vi "AlliGator Source Image ROI Manager.vi"() -> ()   [LabVIEW 2021, in "AlliGator ROIs.lvlib"]
doc: "Source Image ROI list display UI."
uses:
  AlliGator ROIs.lvlib
  AlliGator ROI Manager Actions.ctl
  AlliGator Refnums List.ctl
  Image/Image Control Refnum.ctl
  Image/Image Display Event.ctl
  <vilib>/Utility/miscctls.llb/LVPoint32TypeDef.ctl
  AlliGator Q Element.ctl
  AlliGator Q Event.ctl
  Variant/Variant to Data/Variant to String.vi
  AlliGator Source Image ROI Storage [SGL] v3.vi
  Image/Image.lvlib
  AlliGator Action Engine.lvlib
  Notebook/Notebook.lvlib
  AlliGator Notebook.lvlib
  Variant/Variant to Data/Variant to Data.lvlib
  AlliGator Source Image.lvlib
  AlliGator Globals, Variables & Constants.lvlib
  Rich Text Box/Rich Text Box.lvlib
panel:
  in  "ROI":i32
  out "# ROIs":i32
  in  "ROI List":i32(listbox)
  # "of"
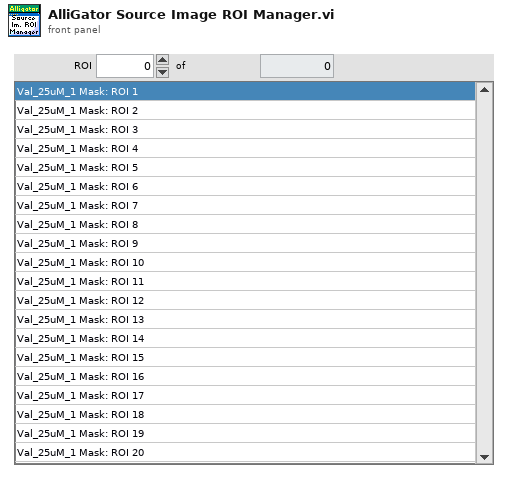
[diagram p1: front panel]
types:
  T1 = typedef "Image.lvlib/Image Control Refnum.ctl" = refnum<vi>
  T2 = typedef "AlliGator Globals, Variables & Constants.lvlib/AlliGator Refnums List.ctl" = enum16{"---------- AlliGator Controls ----------", "AlliGator Tab Control Refnum", "---------- AlliGator Indicators ----------", "Source Image Display Refnum", "Phasor Plot Display Refnum", "Decay Fit Parameter Map Refnum", "---------- AlliGator VIs ----------", "AlliGator Settings Refnum", "AlliGator Launcher Refnum"}
  T3 = typedef "AlliGator ROIs.lvlib/AlliGator ROI Manager Actions.ctl" = enum16{"Undefined", "Delete Current ROI", "Delete All Unselected ROIs", "Delete Multiple ROIs", "Delete All ROIs", "Swap ROIs", "Insert ROI", "Update Current ROI Descriptor", "Rename Current ROI", "Store New ROI", "Store Multiple ROIs", "Select Next ROI", "Select Previous ROI", "Find Selected ROI", "Show All ROIs", "Update ROI Manager Window", "Merge All ROIs", "Unmerge ROI", "Set Selected ROI by ID"}
  T4 = typedef "AlliGator ROIs.lvlib/AlliGator Image ROI Event refnum.ctl" = refnum<user-event>
  T5 = typedef "ROI Descriptor" = cluster{"Global Rectangle":i32[], "Contours":cluster{"ID":enum32{"External", "Internal"}, "Type":u32, "Coordinates":i32[]}[]}
  T6 = typedef "Image.lvlib/Image Display Event.ctl" = cluster{"Item Tag":string, "Image Control Refnum":T1, "Coords":T7, "Item Path":string}
  T7 = typedef "LVPoint32TypeDef.ctl" = cluster{"Horizontal":i32, "Vertical":i32}
  T8 = typedef "AlliGator Action Engine.lvlib/AlliGator Q Element.ctl" = cluster{"AlliGator Q Event":T9, "Data":variant}
  T9 = typedef "AlliGator Action Engine.lvlib/AlliGator Q Event.ctl" = enum16{"---- Files ----", "Files:Set Batch Export Files To Save", "Files:Set Dataset Loading & Pre-processing Options", "Files:Check #Frames in Dataset", "Files:Increment Frame Index", "Files:Open Mask Image", "Files:Open White Light Image", "Files:Open Single Dataset", "Files:New Folder of Folders Selected", "Files:Load File (all Types)_Scriptable", "Files:Move Flattened Series to Folders Series", "Files:Select Folder", "Files:Load FLI Dataset", "Files:Load Swiss SPAD 1 Dataset", "Files:Load Swiss SPAD 2 Dataset", "Files:Load .sdt FLI Dataset", "Files:Load .ptu FLI Dataset", "Files:Load .bin FLI Dataset", "Files:Load Single Gate Image Folder", "Files:Load I/m/phi Dataset (deprecated)", "Files:Load Single Image", "Files:Subtract Background File", "Files:Export FLI Dataset", "Files:Load HDF5 FLI Dataset", "Files:Set Destination File Path", "Files:Save Mask Image", "Files:Batch Conversion", "Files:New Folder Selected", "Files:Close FLI Dataset", "Files:Close FLI Dataset Series", "Files:Close White Light Image", "Files:Close Mask Image", "---- FLI Dataset ----", "FLI Dataset:Channel Arithmetic", "FLI Dataset:Export Average Lifetime Map as ASCII", "FLI Dataset:Export User-Defined Quantity Map as ASCII", "FLI Dataset:Python Function FLI Dataset Event", "FLI Dataset:ROI Analysis", "FLI Dataset:Tilted Logistic Square Gated IRF Characteristics Map", "FLI Dataset:Logistic Square Gated IRF Characteristics Map", "FLI Dataset:Square Gated IRF Characteristics Map", "FLI Dataset:Multi-ROI Single-Pixel Phasor Analysis", "FLI Dataset:Multi-ROI Single-Pixel NLSF Analysis", "FLI Dataset:All ROIs IRF Extraction", "FLI Dataset:All ROIs Decay Fit Non-Interactive (Fast + Individual IRF)", "FLI Dataset:All ROIs Phasor Analysis", "FLI Dataset:All ROIs Decay Fit", "FLI Dataset:Fluorescence Decay Statistics", "FLI Dataset:Update Decay Statistics Graph", "FLI Dataset:Get Decay from ROI", "FLI Dataset:All ROIs Average Lifetimes", "---- FLI Dataset Series ----", "FLI Dataset Series:Sum All Datasets in Series", "FLI Dataset Series:Add Dataset to Accumulated Dataset", "FLI Dataset Series:Display Accumulated Dataset", "FLI Dataset Series:Clear Dataset Series Sum", "FLI Dataset Series:Time-Series Analysis (NLSF)", "FLI Dataset Series:Time-Series Analysis (Phasor)", "---- Image ----", "Image:Update Image Profile Plots", "Image:Image Histogram Cursor Move", "Image:Image Histogram", "Image:Image Contrast", "Image:Set Image Histogram Cursor Move Flag", "Image:Clear Image Overlay", "Image:Use ROI as Search Area", "Image:Set ROI Diameter", "Image:Save Image Data as TIFF", "Image:Save Displayed Image with Overlay", "Image:Save Image Overlay Only", "Image:Save Image as Hot Pixel Mask", "Image:Change Source Image Color Palette", "Image:Copy Image to Clipboard", "Image:Source Image ROI Selection", "Image:Delete All ROIs", "Image:Delete All Unselected ROIs", "Image:Delete ROI", "Image:Merge All ROIs", "Image:Store ROI", "Image:Source Image ROI Storage", "Image:Export ROI Description to Notebook", "Image:Save ROI", "Image:Load ROI", "Image:Paste ROI Definition", "Image:Clear ROI", "Image:Identify ROIs in Mask Image", "Image:Create Complementary ROI", "Image:Create Contour ROI", "Image:Create ROI(s) from Pixels with Peak above Min_Scriptable", "Image:Create ROI(s) from Pixels with Intensity above Min_Scriptable", "Image:Compute ROI Statistics", "Image:Delete ROI(s) based on ROI Characteristics", "Image:Create ROI Grid", "Image:ROI to Individual Pixel ROIs", "Image:Python Function Source Image Event", "Image:Show Phasor Calibration Map ROI Centers", "Image:Convert ROI to Mask Image", "Image:Mouse Move", "Image:Mouse Up", "Image:Set Source Image Mouse Move Flag", "Image:Add Scale Bar Overlay", "Image:Delete Existing ROIs Option", "---- Decay ----", "Decay:Clear IRF/Reference Plot", "Decay:Clear Local IRFs", "Decay:Add Decay to Graph", "Decay:Smoothen Plot", "Decay:Smoothen Plot Tail", "Decay:Average Selected Plots", "Decay:Extract IRF", "Decay:Optimal IRF Extraction", "Decay:Threshold IRF", "Decay:Fit to Model IRF", "Decay:Fit IRF to Square Gate", "Decay:Fit IRF to Logistic Square Gate", "Decay:Fit IRF to Tilted Logistic Square Gate", "Decay:Create Bounding Cursors Set", "Decay:Export Bounding Cursors Definition to Notebook", "Decay:Denoise Plot", "Decay:Compute Cumulative Function", "Decay:Use as Reference Decay", "Decay:Show Reference Decay/IRF", "Decay:Extrapolate Decay", "Decay:Create Head & Tail Bounding Cursors", "Decay:Store Cursor-defined Head & Tail Fractions", "Decay:Rebin Plot", "Decay:1-Normalize Decay", "Decay:[0-1]-Normalize Plot", "Decay:Straighten Decay", "Decay:Shift Decay", "Decay:Fold Decay", "Decay:Fit Decay", "Decay:Global Fit of Selected Decays", "Decay:Post Global Fit Script", "Decay:Add Global Fit Parameters to Graph", "Decay:Add Decay Parameter(s) to Plot (Graph)", "Decay:Export Decay to Phasor Graph", "Decay:Plot Decay Shifts", "Decay:Compute Average Lifetime", "Decay:Plot Convolution", "Decay:Graph Tip Strip Update", "---- Decay Statistics ----", "Decay Statistics:Tip Strip Update", "---- Intensity Time Trace ----", "Intensity Time Trace:Use File Timestamp", "Intensity Time Trace:Load Intensity Corrections File", "Intensity Time Trace:Clear Intensity Corrections File", "Intensity Time Trace:Tip Strip Update", "---- Phasor Plot ----", "Phasor Plot:Build Phasor Plot", "Phasor Plot:Change Phasor Plot Color Palette", "Phasor Plot:Adjust Phasor Plot Display Range", "Phasor Plot:Highlight Image ROI in Phasor Plot", "Phasor Plot:Save Phasor Plot Image with Overlay", "Phasor Plot:Export Complex Phasor Map", "Phasor Plot:Export Phasor Ratio Map", "Phasor Plot:Export Average Lifetime Map", "Phasor Plot:Compute Phase Lifetime Histogram", "Phasor Plot:Compute Phasor Ratio Histogram", "Phasor Plot:Compute Phase Lifetime vs Intensity Scatter Plot", "Phasor Plot:Weber 2-Component Decomposition", "Phasor Plot:Update Phasor Color Map Vertices", "Phasor Plot:Clear Phasor Overlay", "Phasor Plot:Use Segment Extremities as References", "Phasor Plot:Use UC/Segment Intersections as References", "Phasor Plot:Use UC/Principal Axis Intersections as References", "Phasor Plot:Use UC/Linear Fit Intersections as References", "Phasor Plot:Update Phasor Plot Reference", "Phasor Plot:Show Local Phasor Info in Phasor Plot", "Phasor Plot:Update Phasor Plot State", "Phasor Plot:Phasor Plot ROI Storage", "Phasor Plot:Phasor Plot ROI Selection", "Phasor Plot:Python Function Phasor Plot Event", "Phasor Plot:Overlay Phasor ROI, Ratio or Map in Source Image", "Phasor Plot:Compute Decay of Selected Phasors", "Phasor Plot:Phasor at Image Pixel", "Phasor Plot:Mouse Move", "Phasor Plot:Mouse Up", "Phasor Plot:Display Range Mouse Move", "Phasor Plot:Set Mouse Move Flag", "---- Phasor Graph ----", "Phasor Graph:Calibrated Phasor Map Series", "Phasor Graph:Whole Image Phasor Scatter Plot (Todo)", "Phasor Graph:Get Phasor Value", "Phasor Graph:Create New Phasor Plot Dialog", "Phasor Graph:Update Last Phasor Value", "Phasor Graph:Update Phasor (m, phi)", "Phasor Graph:Remove Single Phasor from Plot", "Phasor Graph:Add Single Phasor to Plot", "Phasor Graph:Remove Phasor Plot", "Phasor Graph:Remove Selected Phasor Plots", "Phasor Graph:Clear Phasor Data", "Phasor Graph:Clear Phasor Graph", "Phasor Graph:Cursor Move", "Phasor Graph:Draw Cursor Connecting Line", "Phasor Graph:Clear Cursor Connecting Line", "Phasor Graph:Find UC Intersection", "Phasor Graph:Use UC/Cursor-Defined Line Intersections", "Phasor Graph:Use Selected Plots Fitted Line/UC Intersections", "Phasor Graph:Use Selected Plots Principal Axis/UC Intersections", "Phasor Graph:Show Single Phasor", "Phasor Graph:Save Single Phasor Plot", "Phasor Graph:Save All Phasor Plots", "Phasor Graph:Load Phasor Plot(s)", "Phasor Graph:Phasor Multiplication", "Phasor Graph:Compute Average Phasor", "Phasor Graph:Compute Multiple Average Phasors (Selected Plots)", "Phasor Graph:Export Single Phasor Plot Phase Lifetimes", "Phasor Graph:Phase Lifetime Trajectory", "Phasor Graph:Phase Lifetime vs Intensity Scatter Plot (deprecated)", "Phasor Graph:Parameter 2 vs Parameter 1 Scatter Plot", "Phasor Graph:Use Cursor n Location", "Phasor Graph:Set Reference n to Current Phase Lifetime Value", "Phasor Graph:Set Reference n to Lifetime Value", "Phasor Graph:Set Cursor n Location", "Phasor Graph:Save Phasor Graph Image", "Phasor Graph:Update SEPL Plot", "Phasor Graph:Export Single Phasor Plot Data", "Phasor Graph:Export Selected Phasor Plots Data", "Phasor Graph:Python Function Phasor Graph Event", "Phasor Graph:Tip Strip Update", "---- Calibration ----", "Calibration:Set Calibration Type", "Calibration:Load/Save Phasor Calibration", "Calibration:Load/Save Phasor Calibration Series", "Calibration:Load/Save Phasor Calibration Map", "Calibration:Use as Calibration", "Calibration:Compute Optimal Calibration from Phasor References", "Calibration:Clear Phasor Calibration", "Calibration:Single Phasor Calibration Information", "Calibration:Use as Calibration Series", "Calibration:Use as Calibration Map", "Calibration:Clear Calibration Series", "Calibration:Phasor Calibration Series Information", "Calibration:Clear Calibration Map", "Calibration:Phasor Calibration Map Information", "Calibration:Apply Phasor Calibration", "Calibration:Update Single Plot Calibration", "Calibration:Update Multiple Plots Calibration", "Calibration:Clear Single Plot Calibration", "Calibration:Clear All Plots Calibrations", "Calibration:Clear Plot(s) Calibration(s)?", "Calibration:Phasor Calibration Maps (# Gates Series)", "---- Phasor Ratio ----", "Phasor Ratio:Clear Reference n", "Phasor Ratio:Toggle Selected Plot(s)  Lock to Reference 1", "Phasor Ratio:Use as Reference n", "Phasor Ratio:Send Reference n to Notebook", "Phasor Ratio:Toggle Selected Plot(s)  Lock to Reference 2", "Phasor Ratio:Compute Phasor Ratio at Mouse Location", "Phasor Ratio:Compute Phasor Plot's Average Phasor Ratio", "Phasor Ratio:Compute Time-Series Phasor Ratios", "Phasor Ratio:Fit Line to Phasor Ratio Plot", "Phasor Ratio:Save References", "Phasor Ratio:Load References", "Phasor Ratio:Update Phasor Reference 1", "Phasor Ratio:Update Phasor Reference 2", "Phasor Ratio:Move Cursor n to Reference n", "Phasor Ratio:Use as Phasor Reference 1 Lifetime", "Phasor Ratio:Use as Phasor Reference 2 Lifetime", "Phasor Ratio:Export Phasor Ratio Map as ASCII", "Phasor Ratio:Tip Strip Update", "---- Lifetime & Other Parameters Graph ----", "Lifetime:Tip Strip Update", "---- Decay Fit Parameter Map ----", "Decay Fit Parameter Map:Export ROI NLSF Data as ASCII", "Decay Fit Parameter Map:Set Decay Fit  Parameter Map Selection", "Decay Fit Parameter Map:Build Decay Fit Parameter Map", "Decay Fit Parameter Map:Change Decay Fit Parameter Map Color Palette", "Decay Fit Parameter Map:Export Decay Fit Parameter Map Data as ASCII", "Decay Fit Parameter Map:Export All Decay Fit Parameter Maps Data as ASCII", "Decay Fit Parameter Map:Send Map Data to Lifetime Graph", "Decay Fit Parameter Map:Save Decay Fit Parameter Map Image", "Decay Fit Parameter Map:Save-Load IRFs & Fit Data", "Decay Fit Parameter Map:Update Local Decay Plots", "Decay Fit Parameter Map:Python Function Decay Fit Parameters Map Event", "Decay Fit Parameter Map:Overlay Decay Fit Parameter Map in Source Image", "Decay Fit Parameter Map:Plot Map Data vs Intensity", "Decay Fit Parameter Map:Mouse Up", "Decay Fit Parameter Map:Display Range Mouse Move", "---- Generic Graph ----", "Generic Graph:Generic XY Graph Event", "Generic Graph:Python Function XY Graph Event", "Generic Graph:New Plot", "Generic Graph:Save Plot", "Generic Graph:XY Plot Histogram", "Generic Graph:Set XY Graph Plot Name", "Generic Graph:Set Last Cursor Style", "Generic Graph:Tip Strip Update", "---- GUI ----", "GUI:Start Script", "GUI:Type of Displayed Image Changed", "GUI:Gate Image Slide Changed", "GUI:Show Busy Icon", "GUI:Show Busy Icon & Abort Button", "GUI:Hide Busy Icon", "GUI:Hide Busy Icon & Abort Button", "GUI:Abort", "GUI:End Script", "GUI:Start Timing", "GUI:End Timing", "GUI:Set State Indicator", "GUI:Send Parameters JSON Strings to Clipboard", "GUI:Set Gate Step", "GUI:Idle", "GUI:Initialization", "GUI:Quit", "GUI:Increment Dataset Index", "GUI:Set Dataset Index to -1", "GUI:Time Series Slider Moved", "GUI:Time Series Slider Changed", "GUI:Toggle Playback or Loop", "GUI:Playback Script", "GUI:Set Phasor Frequency", "GUI:Open Window", "GUI:Start Test Script", "GUI:End Test Script", "DEBUG"}
  T10 = cluster{"data name":string, "drag data":variant}[]
  T11 = typedef "Image.lvlib/Named ROI Description.ctl" = cluster{"ROI Descriptor":T5, "ROI Name":string, "Overlay Color":u32}
  T12 = typedef "Rich Text Box.lvlib/Text Formatting.ctl" = cluster{"Font":string, "Text Color":T13, "Text Background Color":T13, "Text Style":enum16{"Regular", "Bold", "Italic", "Underline", "Strikeout"}, "Font Size (Points)":dbl, "Text Alignment":i32}
  T13 = typedef "Rich Text Box.lvlib/Text Colors.ctl" = enum16{"Unchanged", "Black", "Blue", "Brown", "Gray", "Green", "Orange", "Pink", "Red", "White"}
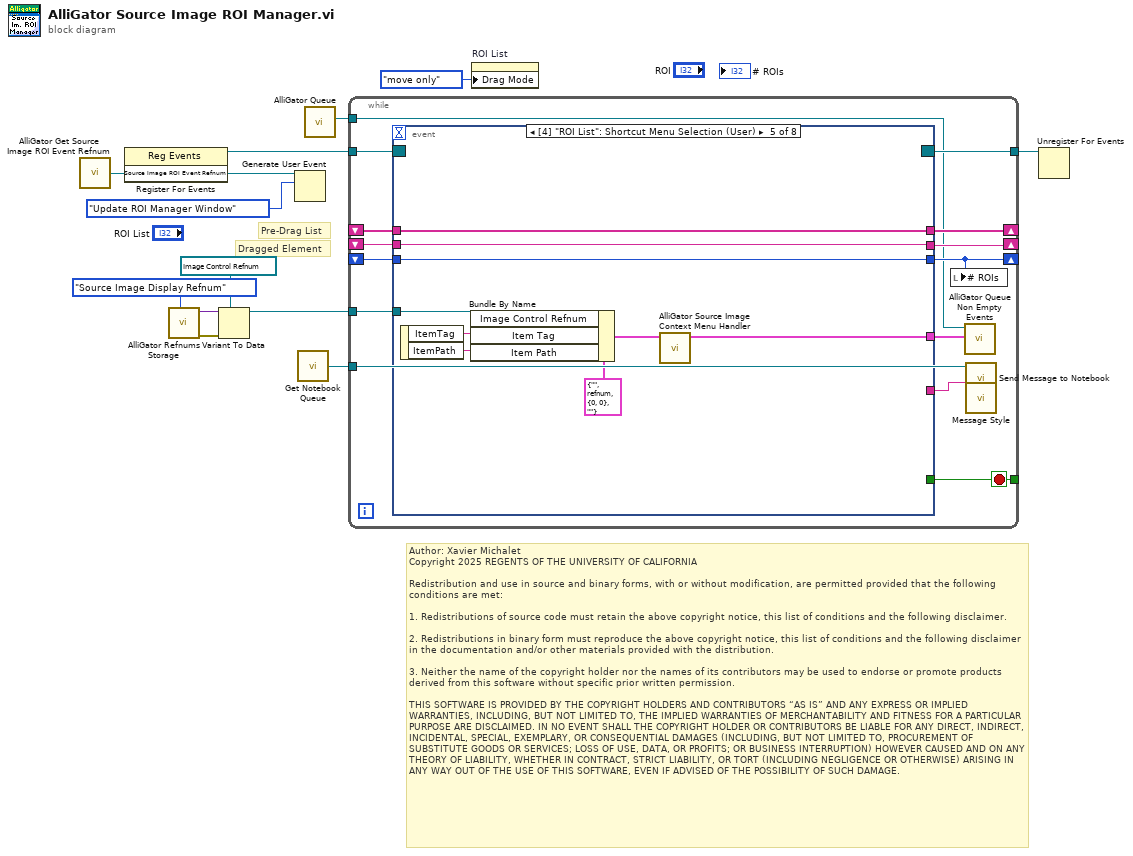
[diagram p0: block diagram]
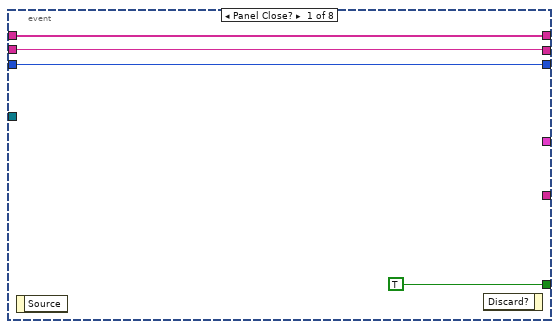
[diagram p2: hidden frame]
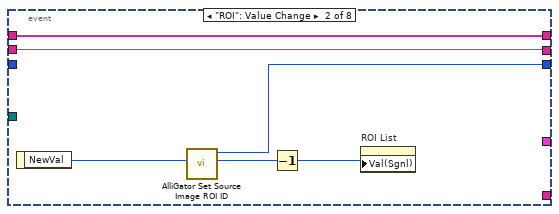
[diagram p3: hidden frame]
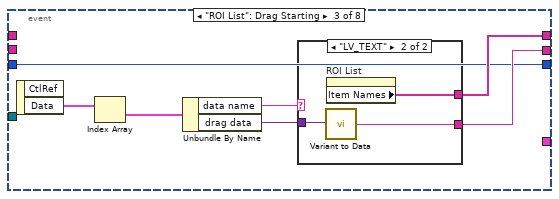
[diagram p4: hidden frame]
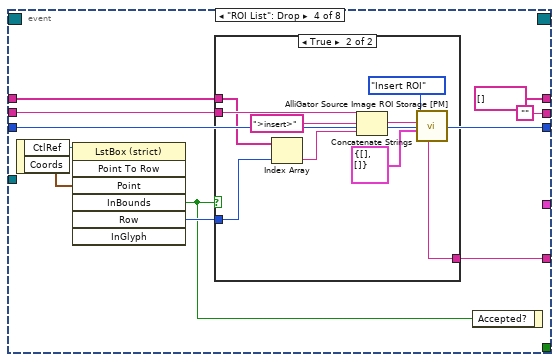
[diagram p6: hidden frame]
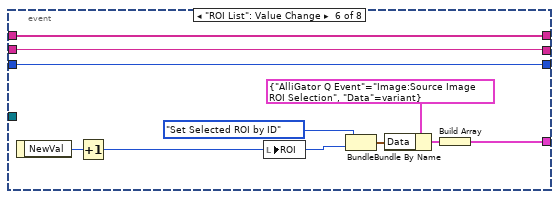
[diagram p8: hidden frame]
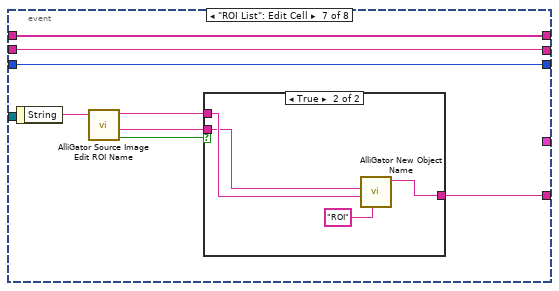
[diagram p9: hidden frame]
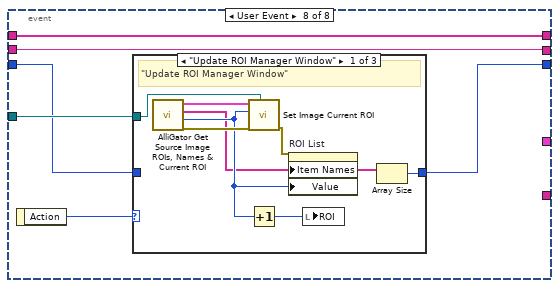
[diagram p11: hidden frame]
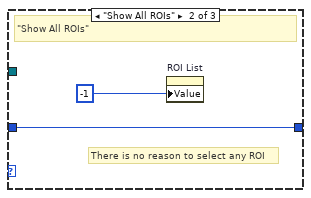
[diagram p12: hidden frame]
diagram:
  # "Author: Xavier Michalet\nCopyright 2025 REGENTS OF THE UNIVERSITY OF CALIFORNIA\n\nRedistribution and use in source and binary forms, with or without modification, are permitted provided that the following conditions are met:\n\n1. Redistributions of source code must retain the above copyright notice, this list of conditions and the following disclaimer.\n\n2. Redistributions in binary form must reproduce the above copyright notice, this list of conditions and the following disclaimer in the documentation and/or other materials provided with the distribution.\n\n3. Neither the name of the copyright holder nor the names of its contributors may be used to endorse or promote products derived from this software without specific prior written permission.\n\nTHIS SOFTWARE IS PROVIDED BY THE COPYRIGHT HOLDERS AND CONTRIBUTORS “AS IS” AND ANY EXPRESS OR IMPLIED WARRANTIES, INCLUDING, BUT NOT LIMITED TO, THE IMPLIED WARRANTIES OF MERCHANTABILITY AND FITNESS FOR A PARTICULAR PURPOSE ARE DISCLAIMED. IN NO EVENT SHALL THE COPYRIGHT HOLDER OR CONTRIBUTORS BE LIABLE FOR ANY DIRECT, INDIRECT, INCIDENTAL, SPECIAL, EXEMPLARY, OR CONSEQUENTIAL DAMAGES (INCLUDING, BUT NOT LIMITED TO, PROCUREMENT OF SUBSTITUTE GOODS OR SERVICES; LOSS OF USE, DATA, OR PROFITS; OR BUSINESS INTERRUPTION) HOWEVER CAUSED AND ON ANY THEORY OF LIABILITY, WHETHER IN CONTRACT, STRICT LIABILITY, OR TORT (INCLUDING NEGLIGENCE OR OTHERWISE) ARISING IN ANY WAY OUT OF THE USE OF THIS SOFTWARE, EVEN IF ADVISED OF THE POSSIBILITY OF SUCH DAMAGE."
  # "Dragged Element"
  # "Pre-Drag List"
  n1 = call "AlliGator Get Source Image ROI Event Refnum.vi"() -> ("Source Image ROI Event Refnum"=w8:T4)
  n2 = register-events(w8) -> (reference out=w12:refnum<event-registration>)  [unwired: 2 in, 1 out]
  n3 = call "AlliGator Refnums Storage.vi"("AlliGator Refnum List"=AlliGator_Refnums_List."Source Image Display Refnum") -> ("Error Out"=w6:errorcluster, "Data out"=w5:variant)  [unwired: 9 in]
  n4 = Variant To Data(error in=w6, type=T1 refnum ("Image Control Refnum"), Variant=w5) -> (data=w3:T1)  [unwired: 1 out]
  n5 = Generate User Event(user event=w8, event data cluster=AlliGator_ROI_Manager_Actions."Update ROI Manager Window" ("Action")) -> ()  [unwired: 2 in, 2 out]
  n6 = call "Get Notebook Queue.vi"() -> ("Notebook Queue"=w9:refnum<queue>)  [unwired: 9 in]
  n7 = call "AlliGator Queue.vi"() -> ("AlliGator Q"=w10:refnum<queue>)  [unwired: 8 in, 1 out]
  n8 = while {
    tunnel: w12 -> [w27]
    tunnel: [w26] -> w11
    tunnel: w10 -> [w16]
    tunnel: w9 -> [w14]
    shift-right: [w25] -> _
    shift-left: _ -> [w24]
    shift-right: [w23] -> _
    shift-left: _ -> [w22]
    tunnel: w3 -> [w21]
    shift-right: [w19] -> _
    shift-left: _ -> [w20]
    tunnel: [w18] -> _
    stop <- w18 stop-if-true
    n9 = event shown="[4] \"ROI List\": Shortcut Menu Selection (User)" {
      selector: w27 -> [_ _ _ _ _ _ _ _]
      dyn-events: [_ _ _ _ _ _ _ _] -> w26
      timeout: _ -> [_ _ _ _ _ _ _ _]
      tunnel: [TRUE _ _ _ _ _ _ _] -> w18
      tunnel: [w30 w37 w41 "" ("String") w75 w85 w90 w103] -> w25
      tunnel: w24 -> [w30 w37 _ w57 w75 w85 w90 w103]
      tunnel: [w29 w36 w39 string[] [] ("Item Names") w74 w84 w89 w102] -> w23
      tunnel: w22 -> [w29 w36 _ w56 w74 w84 w89 w102]
      tunnel: w21 -> [_ _ _ _ w69 _ _ w100]
      tunnel: w20 -> [w28 _ w38 w53 w73 w82 w87 w98]
      tunnel: [w28 w35 w38 w53 w73 w82 w87 w99] -> w19
      tunnel: [_ _ _ _ w67 w76 _ _] -> w17
      tunnel: [_ _ _ w48 _ _ w86 _] -> w13
      event Panel Close? {
        n10 = event-data() -> ()  [unwired: 1 in, 1 out]
        n11 = event-data() -> ()  [unwired: 2 in, 1 out]
      }
      event "ROI": Value Change {
        n12 = event-data() -> ("NewVal"=w34:i32)  [unwired: 1 in]
        n13 = call "AlliGator Set Source Image ROI ID.vi"("New ROI ID"=w34) -> ("New ROI ID"=w33:i32, "# ROIs"=w35:i32)  [unwired: 8 in, 1 out]
        n14 = Decrement(x=w33) -> (x-1=w32:i32)
        n15 = property on="ROI List" class="LstBox (strict)"("Val(Sgnl)"=w32) -> ()  [unwired: 2 in, 2 out]
      }
      event "ROI List": Drag Starting {
        n16 = event-data() -> ("Data"=w44:T10)  [unwired: 1 in, 1 out]
        n17 = Index Array(array=w44) -> (element=w43:cluster{"data name":string, "drag data":variant})  [unwired: 1 in]
        n18 = Unbundle By Name(w43) -> ("data name"=w42:string, "drag data"=w40:variant)
        n19 = case shown="\"LV_TEXT\"" w42 {
          tunnel: [_ w46] -> w41
          tunnel: w40 -> [_ w47]
          tunnel: [_ w45] -> w39
          frame "False", Default {
          }
          frame "LV_TEXT" {
            n20 = call-poly "Variant to Data.vi"("Variant"=w47) -> ("String"=w46:string)  [unwired: 8 in]
            n21 = property on="ROI List" class="LstBox (strict)"() -> ("Item Names"=w45:string[])  [unwired: 2 in, 2 out]
          }
        }
      }
      event "ROI List": Drop {
        n22 = event-data() -> ("CtlRef"=w52:refnum<vi>, "Coords"=w51:T7)  [unwired: 1 in]
        n23 = invoke class="LstBox (strict)" method="Point To Row"(reference=w52, "Point"=w51) -> ("InBounds"=w49:bool, "Row"=w50:i32)  [unwired: 5 in, 5 out]
        n24 = case shown="True" w49 {
          tunnel: w57 -> [_ w64]
          tunnel: w56 -> [_ w61]
          tunnel: w50 -> [_ w59]
          tunnel: [_ w58] -> w48
          frame False {
          }
          frame True {
            n25 = Index Array(array=w61, index=w59) -> (element=w60:string)
            n26 = Concatenate Strings(w64, ">insert>" ("string"), w60) -> (w66:string)
            n27 = call-poly "AlliGator Source Image ROI Storage [PM].vi"("Current ROI Descriptor"=T5 {"Global Rectangle"=[], "Contours"=[]}, "Default Name (\"ROI\")"=w66, "Action"=AlliGator_ROI_Manager_Actions."Insert ROI") -> ("Message"=w58:string)  [unwired: 2 in, 6 out]
          }
        }
        n28 = event-data("Accepted?"=w49) -> ()  [unwired: 1 in, 1 out]
      }
      event "ROI List": Shortcut Menu Selection (User) {
        n29 = event-data() -> ("ItemTag"=w71:string, "ItemPath"=w70:string)  [unwired: 1 in]
        n30 = Bundle By Name(cluster=T6 {"Item Tag"="", "Image Control Refnum"=refnum, "Coords"={"Horizontal"=0, "Vertical"=0}, "Item Path"=""} ("Image Event"), "Image Control Refnum"=w69, "Item Tag"=w71, "Item Path"=w70) -> (w68:T6)
        n31 = call "AlliGator Source Image Context Menu Handler.vi"("Image Event Data"=w68) -> ("AlliGator Actions"=w67:T8[])  [unwired: 9 in, 1 out]
      }
      event "ROI List": Value Change {
        n32 = event-data() -> ("NewVal"=w83:i32)  [unwired: 1 in]
        n33 = Increment(x=w83) -> (x+1=w81:i32)
        n34 = local write "ROI"(w81) -> ()
        n35 = Bundle("Action"=AlliGator_ROI_Manager_Actions."Set Selected ROI by ID", w81) -> (w77:cluster{"Action":T3, i32})  [unwired: 1 in]
        n36 = Bundle By Name(cluster=T8 {"AlliGator Q Event"=enum."Image:Source Image ROI Selection", "Data"=variant} ("element"), "Data"=w77) -> (w79:T8)
        n37 = Build Array(w79) -> (w76:T8[])
      }
      event "ROI List": Edit Cell {
        n38 = event-data() -> ("String"=w93:string)  [unwired: 1 in]
        n39 = call "AlliGator Source Image Edit ROI Name.vi"("ROI Name in"=w93) -> ("accepted?"=w91:bool, "old ROI Name"=w88:string, "ROI Name out"=w92:string)  [unwired: 8 in]
        n40 = case shown="True" w91 {
          tunnel: w92 -> [_ w97]
          tunnel: w88 -> [_ w96]
          tunnel: [_ w94] -> w86
          frame False {
          }
          frame True {
            n41 = call "AlliGator New Object Name.vi"("Object String ('ROI')"="ROI", "Modified Object Name"=w97, "Original Object Name"=w96) -> ("Message"=w94:string)  [unwired: 7 in, 1 out]
          }
        }
      }
      event User Event {
        n42 = event-data() -> ("Action"=w101:T3)  [unwired: 1 in]
        n43 = case shown="\"Update ROI Manager Window\"" w101 {
          tunnel: w100 -> [w109 _ _]
          tunnel: [w105 w112 w114] -> w99
          tunnel: w98 -> [_ w112 w114]
          frame "Update ROI Manager Window" {
            # "\"Update ROI Manager Window\""
            n44 = call "AlliGator Get Source Image ROIs, Names & Current ROI.vi"() -> ("Error Out"=w110:errorcluster, "Current ROI"=w107:i32, "ROI Names"=w106:string[], "Stored ROIs"=w111:T11[])  [unwired: 8 in]
            n45 = call "Set Image Current ROI.vi"("Image Refnum"=w109, "error in (no error)"=w110, "Current ROI"=w107, "Stored ROIs in"=w111) -> ("Error Out"=w108:errorcluster)  [unwired: 7 in]
            n46 = Increment(x=w107) -> (x+1=w104:i32)
            n47 = property on="ROI List" class="LstBox (strict)"(error in=w108, "Item Names"=w106, "Value"=w107) -> ()  [unwired: 1 in, 2 out]
            n48 = local write "ROI"(w104) -> ()
            n49 = Array Size(array=w106) -> (size(s)=w105:i32)
          }
          frame "Show All ROIs" {
            # "There is no reason to select any ROI"
            # "\"Show All ROIs\""
            n50 = property on="ROI List" class="LstBox (strict)"("Value"=-1 ("ROI List")) -> ()  [unwired: 2 in, 2 out]
          }
          frame Default {
          }
        }
      }
    }
    n51 = local write "# ROIs"(w19) -> ()
    n52 = call "AlliGator Queue Non Empty Events.vi"("Actions"=w17, "AlliGator Q"=w16) -> ()  [unwired: 9 in, 1 out]
    n53 = call "Message Style.vi"() -> ("Message Formatting"=w15:T12)
    n54 = call "Send Message to Notebook.vi"("Text Formatting"=w15, "Message"=w13, "Notebook Queue"=w14) -> ()  [unwired: 5 in, 2 out]
  }
  n55 = property on="ROI List" class="LstBox (strict)"("Drag Mode"=enum32{"copy or move", "copy only", "move only"}."move only" ("Drag/Drop:Drag Mode")) -> ()  [unwired: 2 in, 2 out]
  n56 = Unregister For Events(event registration refnum=w11) -> ()  [unwired: 1 in, 1 out]
